vi "demo.vi"() -> ()   [LabVIEW 2013]
panel:
  out "相等":bool
  out "面积":dbl[](array[numeric])
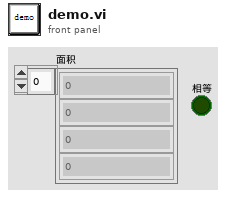
[diagram p1: front panel]
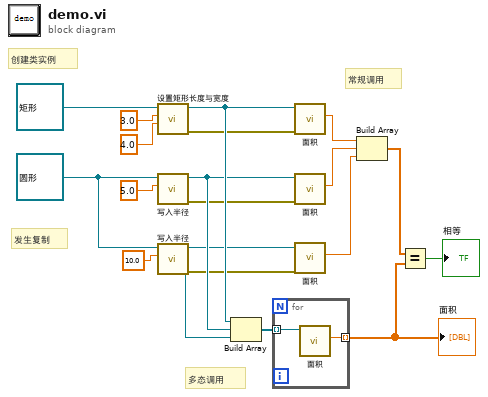
[diagram p0: block diagram]
diagram:
  w16 = refnum<class "圆形.lvclass"> refnum ("圆形.lvclass")
  # "创建类实例"
  # "发生复制"
  # "常规调用"
  # "多态调用"
  n1 = call "设置矩形长度与宽度.vi"("宽度"=4.0, "长度"=3.0, "矩形类 输入"=refnum<class "矩形.lvclass"> refnum ("矩形.lvclass")) -> ("error out"=w11:errorcluster, "矩形类 输出"=w12:refnum<class "矩形.lvclass">)  [unwired: 7 in]
  n2 = call "写入半径.vi"("半径"=5.0, "圆形输入"=w16) -> ("error out"=w9:errorcluster, "圆形输出"=w10:refnum<class "圆形.lvclass">)  [unwired: 8 in]
  n3 = call "写入半径.vi"("半径"=10.0, "圆形输入"=w16) -> ("error out"=w7:errorcluster, "圆形输出"=w8:refnum<class "圆形.lvclass">)  [unwired: 8 in]
  n4 = Build Array(w12, w10, w8) -> (w13:refnum<class "封闭形状.lvclass">[])
  n5 = for {
    tunnel: w13 -> [w21] mode=indexing
    tunnel: [w20] -> w2 mode=indexing
    n6 = call-dynamic "面积.vi"("封闭形状 输入"=w21) -> ("面积"=w20:dbl)  [unwired: 8 in, 2 out]
  }
  "面积" <- w2
  n7 = call-dynamic "面积.vi"("error in (no error)"=w11, "矩形类 输入"=w12) -> ("面积"=w6:dbl)  [unwired: 7 in, 2 out]
  n8 = call-dynamic "面积.vi"("error in (no error)"=w9, "圆形 输入"=w10) -> ("面积"=w5:dbl)  [unwired: 7 in, 2 out]
  n9 = call-dynamic "面积.vi"("error in (no error)"=w7, "圆形 输入"=w8) -> ("面积"=w4:dbl)  [unwired: 7 in, 2 out]
  n10 = Build Array(w6, w5, w4) -> (w3:dbl[])
  n11 = Equal?(x=w3, y=w2) -> (x = y?=→"相等":bool)
